vi "Shooter Controller.vi"(8 "error in":errorcluster) -> ()   [LabVIEW 2019]
doc: "This VI executes continuously carrying out the current operation and responding to updates or new operations. It will often contain the timing or control code that is difficult to place directly in TeleOp. This VI generally opens all sensors and motors and isolates the rest of the robot code from knowing how the operations are carried out."
uses:
  <vilib>/Rock Robotics/WPI/Framework/Completion Status.ctl
  Shooter Setpoints.ctl
  Shooter Operations.ctl
  <vilib>/Rock Robotics/WPI/ThirdParty/Phoenix-LabVIEW/Motor Controller/Controls/CTRE_Phoenix_MotorControl_ControlMode.ctl
  Framework/Robot Global Data.vi
  <vilib>/Rock Robotics/Network Tables/NT Write Number.vi
panel:
  in  "Interactive Values":T1
  out "Current\nCmd":string
  in  "Buttons":cluster{"Execute Cmd":bool, "Abort Cmd":bool}
  out "Command Timing":cluster{"Start Time (ms)":u32, "Iterations":i32}
  out "Status":T3
  # "Tip: It may be helpful to observe inputs and sensor values.\nYou may also want to display tuning or debugging controls."
  # "Interactive Command: You may fill in the settings for a command\nand schedule it with the Execute button. You can observe and abort\nany command while fine tuning the code for the controller."
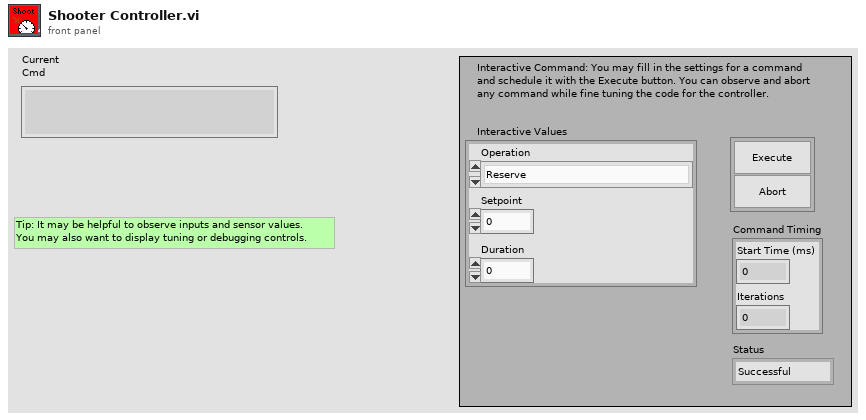
[diagram p1: front panel]
types:
  T1 = typedef "Shooter Setpoints.ctl" = cluster{"Operation":T2, "Setpoint":dbl, "Duration":dbl}
  T2 = typedef "Shooter Operations.ctl" = enum16{"Reserve", "Read Current", "Immediate", "Shooter for Time", "Shooter Immediate"}
  T3 = typedef "Completion Status.ctl" = enum16{"Successful", "Aborted", "Incomplete"}
  T4 = typedef "WPI_MotorControlDeviceRef.ctl" = cluster{"DeviceStatus":errorcluster, "Type":T5, "PWM":cluster{"PWM Channel":T6, "DeadBand":T7}, "CAN":cluster{"Device Number":u8, "SetOutput VI Ref":variant, "GetOutput VI Ref":variant, "Enable VI Ref":variant, "Disable VI Ref":variant, "Data":variant}, "Invert":bool, "DIO PWM":cluster{"PWM \"Enable\" Channel":T6, "DIOChannel":T8, "PWM Rate":dbl}}
  T5 = typedef "WPI_MotorControlType.ctl" = enum16{"PWM", "CAN", "DIO PWM"}
  T6 = typedef "FPGA_DIOPWMChannel.ctl" = enum8{"PWM 0", "PWM 1", "PWM 2", "PWM 3", "PWM 4", "PWM 5", "PWM 6", "PWM 7", "PWM 8", "PWM 9", "PWM MXP 0", "PWM MXP 1", "PWM MXP 2", "PWM MXP 3", "PWM MXP 4", "PWM MXP 5", "PWM MXP 6", "PWM MXP 7", "PWM MXP 8", "PWM MXP 9", "Invalid"}
  T7 = typedef "WPI_PWMDeadband.ctl" = cluster{"Name":string, "maxPositivePwm":i32, "minPositivePwm":i32, "centerPwm":i32, "maxNegativePwm":i32, "minNegativePwm":i32, "angularRange":u16}
  T8 = typedef "FPGA_DIOChannel.ctl" = enum8{"DIO 0", "DIO 1", "DIO 2", "DIO 3", "DIO 4", "DIO 5", "DIO 6", "DIO 7", "DIO 8", "DIO 9", "DIO MXP 0", "DIO MXP 1", "DIO MXP 2", "DIO MXP 3", "DIO MXP 4", "DIO MXP 5", "DIO MXP 6", "DIO MXP 7", "DIO MXP 8", "DIO MXP 9", "DIO MXP 10", "DIO MXP 11", "DIO MXP 12", "DIO MXP 13", "DIO MXP 14", "DIO MXP 15", "SPI Port CS1", "SPI Port CS2", "SPI Port CS3", "SPI Port MISO", "SPI Port MOSI", "Invalid"}
  T9 = typedef "Command Status Info.ctl" = cluster{"Name":string, "Status":T3, "notifier out":T10}
  T10 = typedef "Completion Notifier.ctl" = refnum<notifier>
  T11 = cluster{"Current Command":T1, "Command Timing":cluster{"Start Time (ms)":u32, "Iterations":i32}, "Command Arguments":cluster{"Command Info":T9, "Description":string, "Default Command":T1, "queue out":refnum<queue>, "Subsystem Name":string}}
  T12 = typedef "CTRE_Phoenix_MotorControl_ControlMode.ctl" = u16
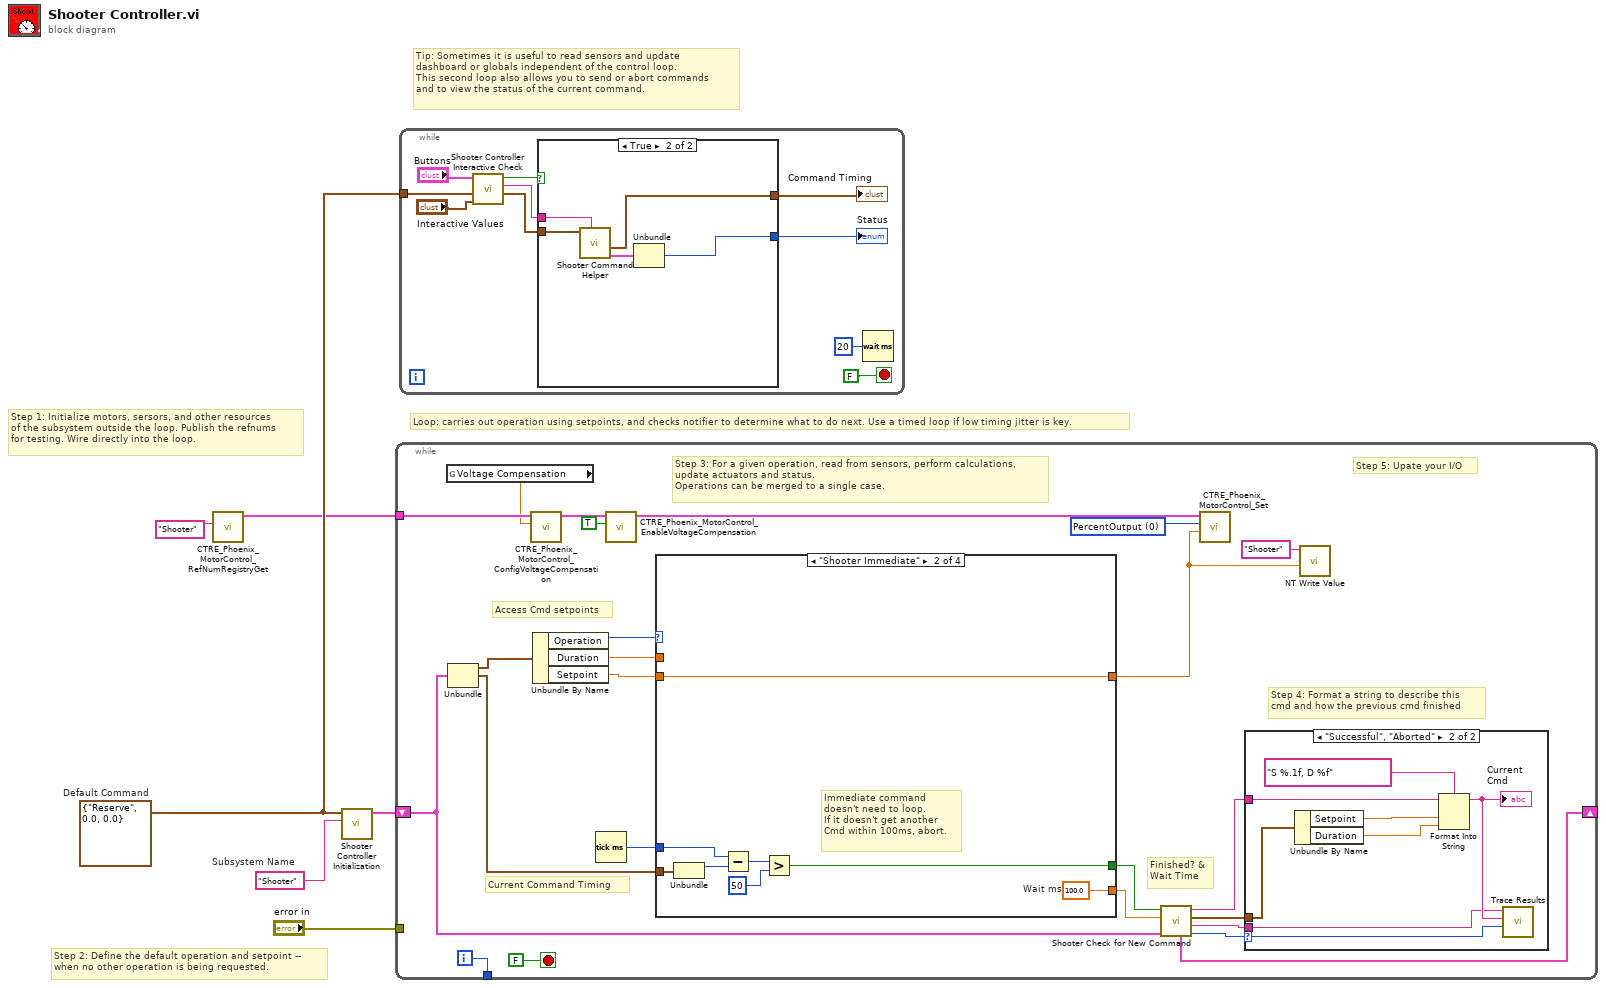
[diagram p0: block diagram]
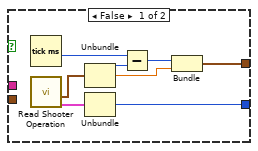
[diagram p2: hidden frame]
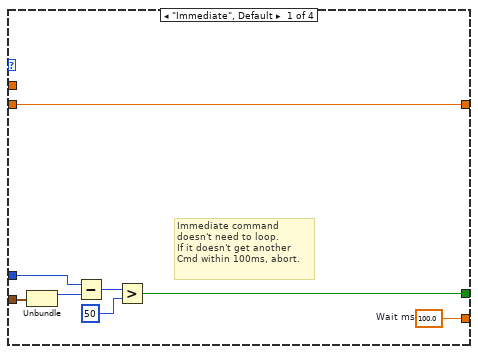
[diagram p4: hidden frame]
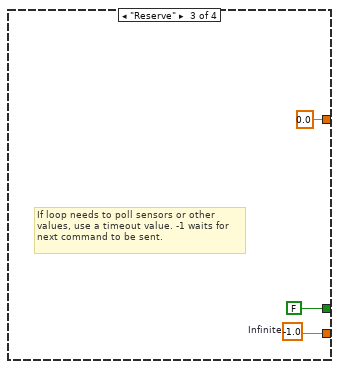
[diagram p5: hidden frame]
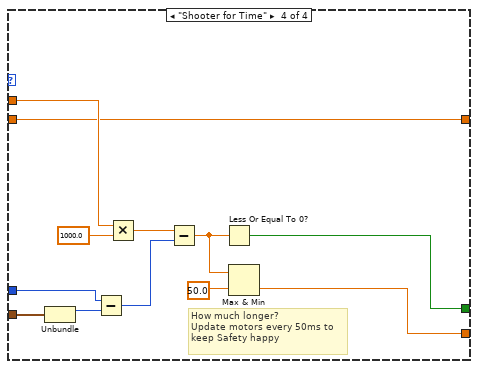
[diagram p6: hidden frame]
diagram:
  w3 = T1 {"Operation"=enum."Reserve", "Setpoint"=0.0, "Duration"=0.0}  # Default Command
  w4 = "Shooter"  # Subsystem Name
  # "Tip: Sometimes it is useful to read sensors and update\ndashboard or globals independent of the control loop.\nThis second loop also allows you to send or abort commands\nand to view the status of the current command."
  # "Step 2: Define the default operation and setpoint --\nwhen no other operation is being requested."
  # "Step 1: Initialize motors, sersors, and other resources\nof the subsystem outside the loop. Publish the refnums\nfor testing. Wire directly into the loop."
  # "Loop: carries out operation using setpoints, and checks notifier to determine what to do next. Use a timed loop if low timing jitter is key."
  n1 = call <vilib>:"CTRE_Phoenix_MotorControl_RefNumRegistryGet.vi"("refnum name"="Shooter") -> ("PhoenixMotorControlDevRef"=w1:T4)  [unwired: 9 in, 1 out]
  n2 = call "Shooter Controller Initialization.vi"("Subsystem Name"=w4, "Default Command"=w3) -> ("Current Command"=w5:T11)  [unwired: 9 in]
  n3 = while {
    shift-right: [w22] -> _
    shift-left: w5 -> [w15]
    tunnel: [w29] -> _
    tunnel: "error in" -> [_]
    tunnel: w1 -> [w10]
    i -> [w29]
    stop <- FALSE stop-if-true
    w14 = T12 0 items=["PercentOutput"=0, "Position"=1, "Velocity"=2, "Current"=3, "Follower"=5, "MotionProfile"=6, "MotionMagic"=7, "MotionProfileArc"=10, "Disabled"=15] ("Control Mode")
    # "Step 5: Upate your I/O"
    # "Step 4: Format a string to describe this\ncmd and how the previous cmd finished"
    # "Current Command Timing"
    # "Access Cmd setpoints"
    # "Finished? &\nWait Time"
    # "Step 3: For a given operation, read from sensors, perform calculations,\nupdate actuators and status.\nOperations can be merged to a single case."
    n4 = global read "Robot Global Data.vi" "Voltage Compensation"() -> (w7:dbl)
    n5 = Unbundle(w15) -> ("Current Command"=w28:T1, "Command Timing"=w24:cluster{"Start Time (ms)":u32, "Iterations":i32})  [unwired: 1 out]
    n6 = call <vilib>:"CTRE_Phoenix_MotorControl_ConfigVoltageCompensation.vi"("Saturation Voltage"=w7, "PhoenixMotorControlDevRef"=w10) -> ("PhoenixMotorControlDevRef"=w11:T4)  [unwired: 8 in, 1 out]
    n7 = Unbundle By Name(w28) -> ("Operation"=w27:T2, "Duration"=w26:dbl, "Setpoint"=w23:dbl)
    n8 = Tick Count (ms)() -> (millisecond timer value=w25:u32)
    n9 = call <vilib>:"CTRE_Phoenix_MotorControl_EnableVoltageCompensation.vi"("Enable Voltage Compensation?"=TRUE, "PhoenixMotorControlDevRef"=w11) -> ("PhoenixMotorControlDevRef"=w9:T4)  [unwired: 8 in, 1 out]
    n10 = case shown="\"Shooter Immediate\"" w27 {
      tunnel: [w46 w54 w57 w59] -> w20
      tunnel: [w40 w48 FALSE ("ignore previous (F)") w58] -> w21
      tunnel: w24 -> [w42 w50 _ w61]
      tunnel: w26 -> [_ _ _ w63]
      tunnel: w25 -> [w41 w49 _ w60]
      tunnel: w23 -> [w39 w47 _ w62]
      tunnel: [w39 w47 0.0 ("Setpoint") w62] -> w13
      frame "Immediate", Default {
        w46 = 100.0  # Wait ms
        # "Immediate command\ndoesn't need to loop.\nIf it doesn't get another\nCmd within 100ms, abort."
        n11 = Unbundle(w42) -> ("Start Time (ms)"=w45:u32)  [unwired: 1 out]
        n12 = Subtract(x=w41, y=w45) -> (x-y=w44:u32)
        n13 = Greater?(x=w44, y=u8 50 ("Left Motor")) -> (0:w40:bool)
      }
      frame "Shooter Immediate" {
        w54 = 100.0  # Wait ms
        # "Immediate command\ndoesn't need to loop.\nIf it doesn't get another\nCmd within 100ms, abort."
        n14 = Unbundle(w50) -> ("Start Time (ms)"=w53:u32)  [unwired: 1 out]
        n15 = Subtract(x=w49, y=w53) -> (x-y=w52:u32)
        n16 = Greater?(x=w52, y=u8 50 ("Left Motor")) -> (0:w48:bool)
      }
      frame "Reserve" {
        w57 = -1.0  # Infinite
        # "If loop needs to poll sensors or other\nvalues, use a timeout value. -1 waits for\nnext command to be sent."
      }
      frame "Shooter for Time" {
        # "How much longer?\nUpdate motors every 50ms to\nkeep Safety happy"
        n17 = Unbundle(w61) -> ("Start Time (ms)"=w67:u32)  [unwired: 1 out]
        n18 = Subtract(x=w60, y=w67) -> (x-y=w64:u32)
        n19 = Multiply(x=w63, y=1000.0) -> (x*y=w65:dbl)
        n20 = Subtract(x=w65, y=w64) -> (x-y=w68:dbl)
        n21 = Less Or Equal To 0?(x=w68) -> (x <= 0?=w58:bool)
        n22 = Max & Min(x=w68, y=50.0) -> (min(x,y)=w59:dbl)  [unwired: 1 out]
      }
    }
    n23 = call "Shooter Check for New Command.vi"("Current Command"=w15, "Wait time (ms)"=w20, "Finished?"=w21) -> ("Completion"=w16:T3, "Subsystem Name"=w17:string, "Current Command"=w18:T1, "Initial Trace String"=w19:string, "NextCommand"=w22:T11)  [unwired: 4 in]
    n24 = call <vilib>:"CTRE_Phoenix_MotorControl_Set.vi"("Output"=w13, "Control Mode"=w14, "PhoenixMotorControlDevRef"=w9) -> ()  [unwired: 7 in, 2 out]
    n25 = case shown="\"Successful\", \"Aborted\"" w16 {
      selector: w16 -> [_ w38]
      tunnel: w19 -> [_ w34]
      tunnel: w18 -> [_ w35]
      tunnel: w17 -> [_ w31]
      frame "Incomplete", Default {
        # "Continuing current command"
      }
      frame "Successful", "Aborted" {
        # "Report and setup for next command"
        n26 = Unbundle By Name(w35) -> ("Setpoint"=w37:dbl, "Duration"=w32:dbl)
        n27 = Format Into String(format string="S %.1f, D %f", initial string=w34, w37, w32) -> (resulting string=w33:string)  [unwired: 1 in, 1 out]
        "Current\nCmd" <- w33
        n28 = call <vilib>:"Trace Results.vi"("Status of previous command"=w38, "Description"=w33, "Subsystem"=w31) -> ()  [unwired: 9 in]
      }
    }
    n29 = call-poly <vilib>:"NT Write Value.vi"("Numeric"=w13, "Name"="Shooter") -> ()  [unwired: 9 in, 1 out]
  }
  n30 = while {
    tunnel: w3 -> [w76]
    stop <- FALSE stop-if-true
    n31 = call "Shooter Controller Interactive Check.vi"("Interactive Command in"="Interactive Values", "Default Command"=w76, "Buttons"="Buttons") -> ("Interactive Command out"=w73:T1, "Trace String"=w74:string, "Schedule"=w75:bool)  [unwired: 6 in]
    n32 = case shown="True" w75 {
      tunnel: [w87 w92] -> w72
      tunnel: w73 -> [_ w90]
      tunnel: [w83 w88] -> w71
      tunnel: w74 -> [_ w91]
      frame False {
        n33 = Tick Count (ms)() -> (millisecond timer value=w82:u32)
        n34 = call "Read Shooter Operation.vi"() -> ("Command Info"=w80:T9, "SubSystem Data"=w81:T1)  [unwired: 9 in, 1 out]
        n35 = Unbundle(w81) -> ("Operation"=w86:T2, "Setpoint"=w84:dbl)  [unwired: 1 out]
        n36 = Unbundle(w80) -> ("Status"=w87:T3)  [unwired: 2 out]
        n37 = Subtract(x=w82, y=w86) -> (x-y=w85:u32)
        n38 = Bundle(w85, "Setpoint"=w84) -> (w83:cluster{u32, "Setpoint":dbl})  [unwired: 1 in]
      }
      frame True {
        n39 = call "Shooter Command Helper.vi"("Description"=w91, "SubSystem Data"=w90) -> ("Command Info Out"=w89:T9, "Command Timing"=w88:cluster{"Start Time (ms)":u32, "Iterations":i32})  [unwired: 7 in, 1 out]
        n40 = Unbundle(w89) -> ("Status"=w92:T3)  [unwired: 2 out]
      }
    }
    "Status" <- w72
    "Command Timing" <- w71
    n41 = Wait (ms)(milliseconds to wait=u32 20) -> ()  [unwired: 1 out]
  }
